vi "Ch1-Ex6.vi"() -> ()   [LabVIEW 2018]
panel:
  out "I":dbl
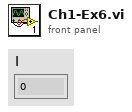
[diagram p1: front panel]
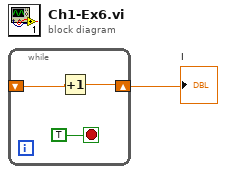
[diagram p0: block diagram]
diagram:
  n1 = while {
    shift-right: [w2] -> w1
    shift-left: _ -> [w3]
    stop <- TRUE stop-if-true
    n2 = Increment(x=w3) -> (x+1=w2:dbl)
  }
  "I" <- w1
